vi "setTargetState.vi"(8 "error in (no error)":errorcluster, 10 "Target State":string, 11 "statemachine in":refnum<class "statemachine.lvclass">) -> (0 "error out":errorcluster, 3 "statemachine out":refnum<class "statemachine.lvclass">)   [LabVIEW 2020, in "eos.lvlib" / "statemachine.lvclass"]
uses:
  statemachine.lvclass
  statemachine.lvclass/statemachine.ctl
  interfaces/state/state.lvclass
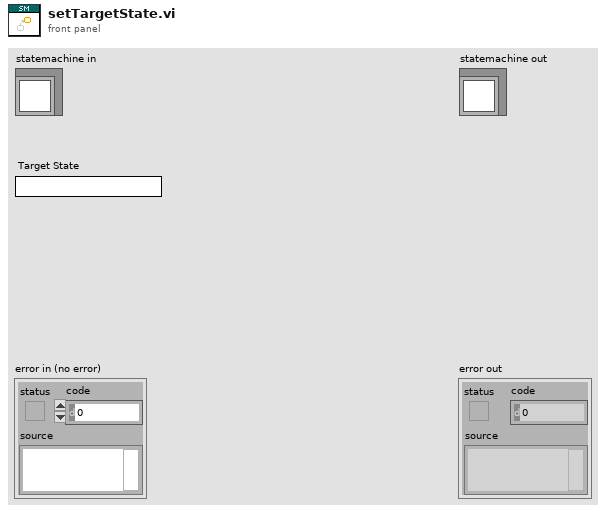
[diagram p1: front panel]
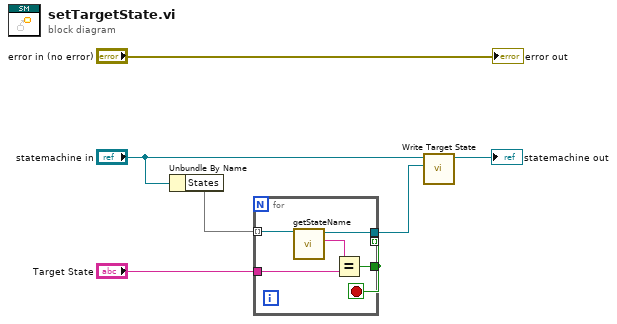
[diagram p0: block diagram]
diagram:
  n1 = Unbundle By Name("statemachine in") -> ("States"=w3:set{refnum<class "state.lvclass">})
  n2 = for {
    tunnel: w3 -> [w11] mode=indexing
    tunnel: "Target State" -> [w9]
    tunnel: [w8] -> w1 if=w7
    tunnel: [w7] -> _ mode=indexing
    tunnel: [w7] -> _
    stop <- w7 stop-if-true
    n3 = call-dynamic "getStateName.vi"("state in"=w11) -> ("State Name"=w10:string, "state out"=w8:refnum<class "state.lvclass">)  [unwired: 8 in, 1 out]
    n4 = Equal?(x=w10, y=w9) -> (x = y?=w7:bool)
  }
  n5 = call "Write Target State.vi"("Target State"=w1, "statemachine in"="statemachine in") -> ("statemachine out"=→"statemachine out":refnum<class "statemachine.lvclass">)  [unwired: 9 in]
  "error out" <- "error in (no error)"
